vi "Configure Signaling TDD DL Slots.vi"(7 "DL Slots (0)":i32, 8 "error in (no error)":errorcluster, 9 "Pattern (1)":T1=1, 10 "Cell Name (\"Cell Name\")":string="Cell Name", 11 "VISA resource name":refnum<visa-resource-name>) -> (0 "error out":errorcluster, 3 "VISA resource name out":refnum<visa-resource-name>)   [LabVIEW 2020, in "Rohde&Schwarz CMWXP NR FR1 Measurement.lvlib"]
doc: "Defines the number of DL slots in the UL-DL pattern <p>.\n\nAttribute:\nRSCMWXPNRFR1M_ATTR_SIGNALING_TDD_DL_SLOTS\n\nRemote-control command:\n[CONFigure:]SIGNaling:NRADio:CELL:TDD:PATTern<p>:DL:NSLots"
uses:
  <instrlib>/Rohde&Schwarz CMWXP NR FR1 Measurement/Rohde&Schwarz CMWXP NR FR1 Measurement.lvlib
  <instrlib>/Rohde&Schwarz CMWXP NR FR1 Measurement/Private/_Pattern.ctl
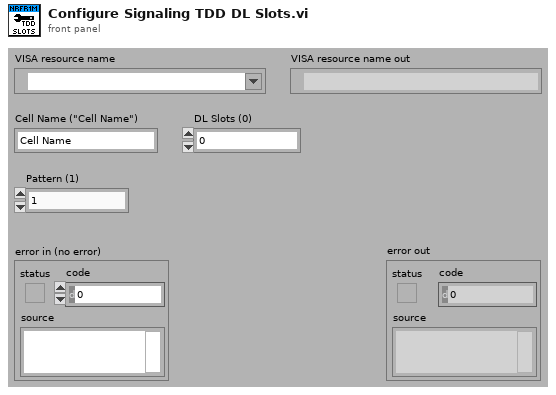
[diagram p1: front panel]
types:
  T1 = typedef "Rohde&Schwarz CMWXP NR FR1 Measurement.lvlib/_Pattern.ctl" = i32
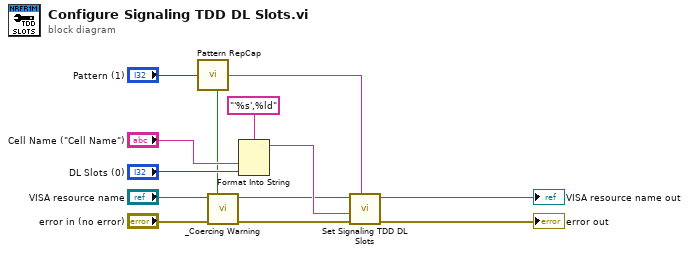
[diagram p0: block diagram]
diagram:
  n1 = call <instrlib>:"Pattern RepCap.vi"("Pattern In"="Pattern (1)") -> ("In Range?"=w1:bool, "RepCap Identifier Out"=w9:string)  [unwired: 1 in]
  n2 = call <instrlib>:"_Coercing Warning.vi"("In Range?"=w1, "error in (no error)"="error in (no error)", "VISA resource name"="VISA resource name") -> ("error out"=w3:errorcluster, "VISA resource name out"=w2:refnum<visa-resource-name>)  [unwired: 7 in]
  n3 = Format Into String(format string="'%s',%ld", "Cell Name (\"Cell Name\")", "DL Slots (0)") -> (resulting string=w8:string)  [unwired: 2 in, 1 out]
  n4 = call "Set Signaling TDD DL Slots"("Repeated Capabilities"=w9, "error in (no error)"=w3, "Signaling TDD DL Slots ()"=w8, "instrument handle"=w2) -> ("error out"=→"error out":errorcluster, "instrument handle out"=→"VISA resource name out":refnum<visa-resource-name>)  [unwired: 6 in]
